vi "TemperatureControl.vi"() -> ()   [LabVIEW 2025]
panel:
  out "Warning":bool
  in  "High Limit":dbl
  out "Temperature History":cluster{dbl, "Thermometer":dbl}(graph)
  in  "Power":bool
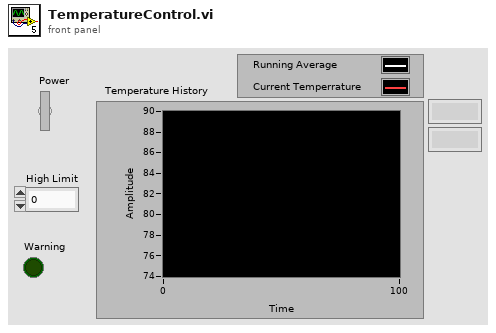
[diagram p1: front panel]
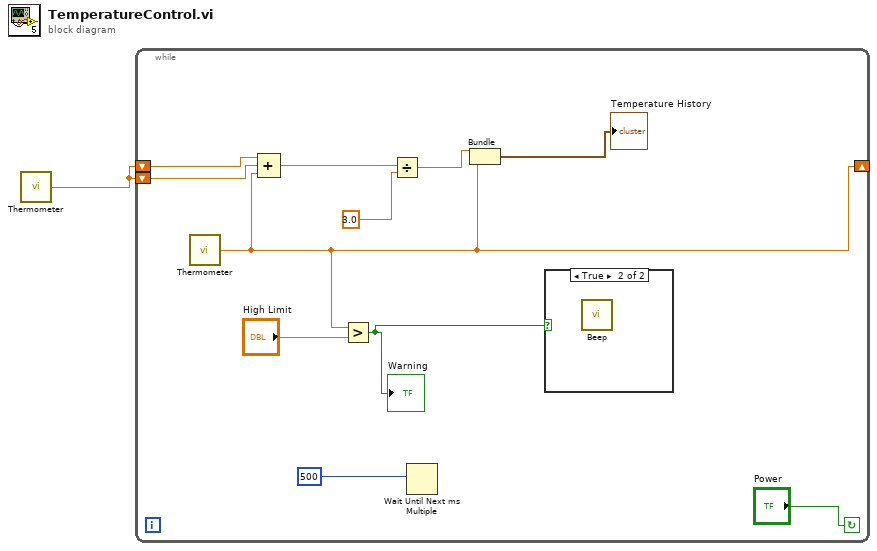
[diagram p0: block diagram]
diagram:
  n1 = call "Thermometer.vi"() -> ("Thermometer"=w1:dbl)  [unwired: 1 in]
  n2 = while {
    shift-right: [w4] -> _
    shift-left: w1 -> [w12]
    shift-left: w1 -> [w11]
    stop <- "Power" continue-if-true
    n3 = call "Thermometer.vi"() -> ("Thermometer"=w4:dbl)  [unwired: 1 in]
    n4 = Compound Arithmetic op=ADD(w12, w11, w4) -> (w10:dbl)
    n5 = Greater?(x=w4, y="High Limit") -> (0:w2:bool)
    "Warning" <- w2
    n6 = Divide(x=w10, y=3.0) -> (x/y=w7:dbl)
    n7 = Wait Until Next ms Multiple(millisecond multiple=500) -> ()  [unwired: 1 out]
    n8 = Bundle(w7, "Thermometer"=w4) -> (→"Temperature History":cluster{dbl, "Thermometer":dbl})  [unwired: 1 in]
    n9 = case shown="True" w2 {
      frame False {
      }
      frame True {
        n10 = call <vilib>:"Beep.vi"() -> ()  [unwired: 12 in]
      }
    }
  }
